vi "Config GUI - Insert Into Virtual Folder.vi"(8 "error in":errorcluster, 10 "Virtual Folder Search Output":T1, 11 "GUI Objects":T2) -> (0 "error out":errorcluster)   [LabVIEW 2022 SP3]
doc: "Configures the GUI objects that play a part in the functionality that inserts the newly created VI or CTL into a Virtual Folder."
uses:
  GUI Objects (cluster).ctl
  DFS Output (cluster).ctl
panel:
  # "Development\ncontrols/indicators useful for development and testing, but which are not outputs of the VI"
  # "Input\nInputs to the VI"
  # "Output\nOutputs of the VI"
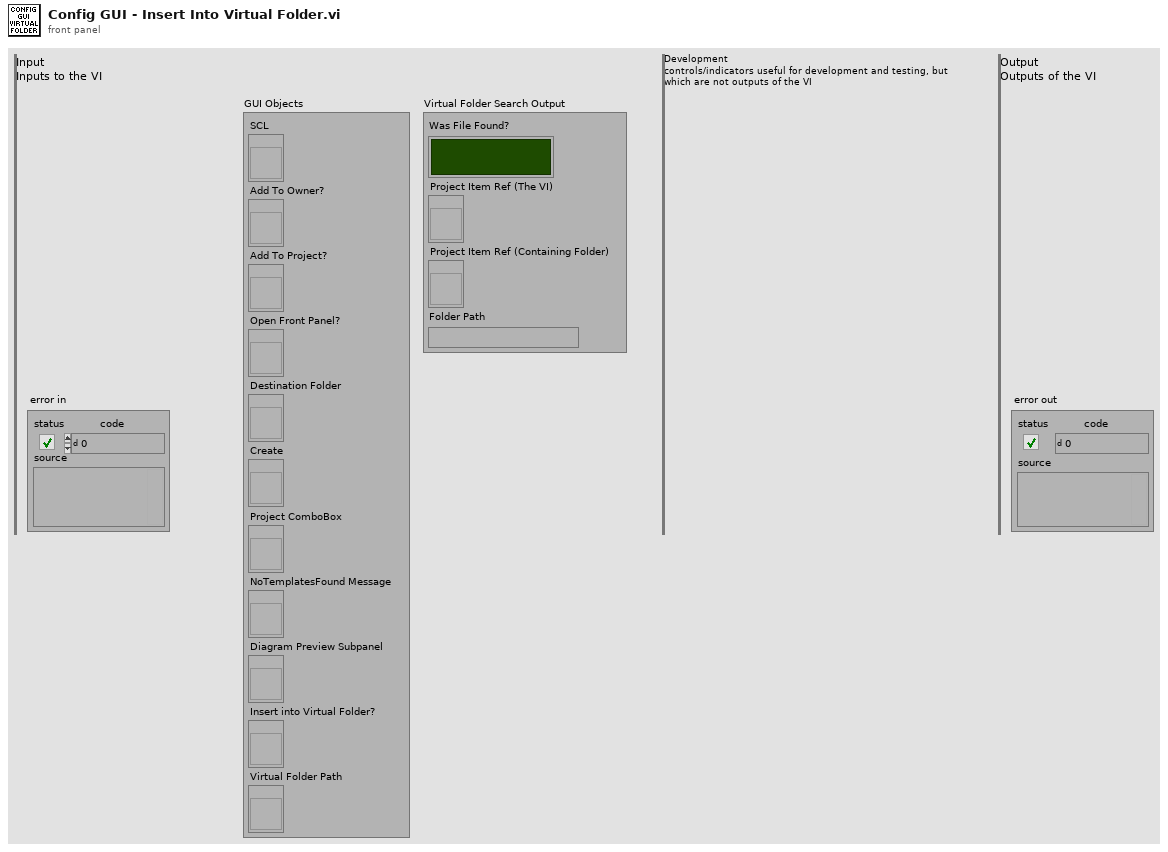
[diagram p1: front panel]
types:
  T1 = typedef "DFS Output (cluster).ctl" = cluster{"Was File Found?":bool, "Project Item Ref (The VI)":refnum<vi>, "Project Item Ref (Containing Folder)":refnum<vi>, "Folder Path":string}
  T2 = typedef "GUI Objects (cluster).ctl" = cluster{"SCL":refnum<vi>, "Add To Owner?":refnum<vi>, "Add To Project?":refnum<vi>, "Open Front Panel?":refnum<vi>, "Destination Folder":refnum<vi>, "Create":refnum<vi>, "Project ComboBox":refnum<vi>, "NoTemplatesFound Message":refnum<vi>, "Diagram Preview Subpanel":refnum<vi>, "Insert into Virtual Folder?":refnum<vi>, "Virtual Folder Path":refnum<vi>}
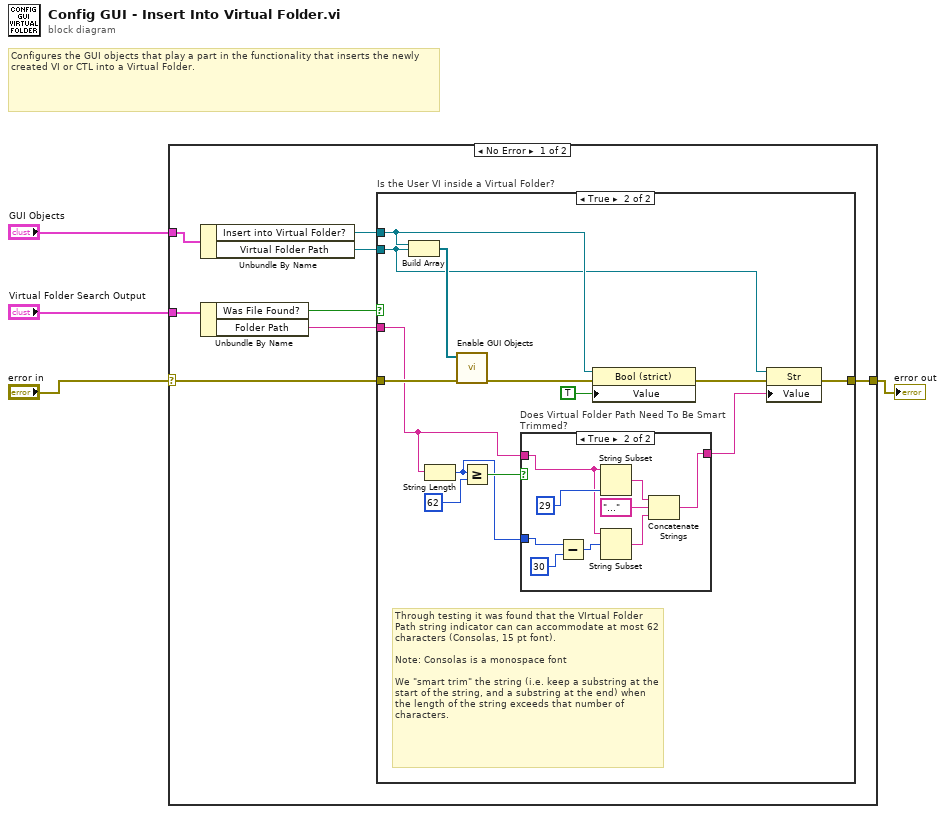
[diagram p0: block diagram]
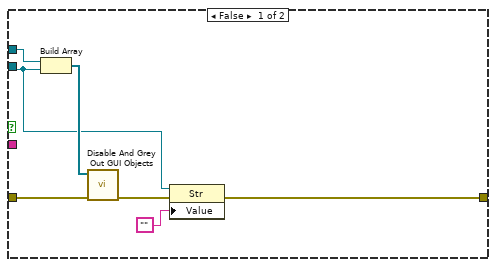
[diagram p2: hidden frame]
diagram:
  # "Configures the GUI objects that play a part in the functionality that inserts the newly created VI or CTL into a Virtual Folder."
  n1 = case shown="No Error" "error in" {
    selector: "error in" -> [w11 w43]
    tunnel: [w10 w43] -> w3
    tunnel: "GUI Objects" -> [w8 _]
    tunnel: "Virtual Folder Search Output" -> [w12 _]
    frame No Error {
      n2 = Unbundle By Name(w8) -> ("Insert into Virtual Folder?"=w7:refnum<vi>, "Virtual Folder Path"=w6:refnum<vi>)
      n3 = Unbundle By Name(w12) -> ("Was File Found?"=w9:bool, "Folder Path"=w5:string)
      n4 = case "Is the User VI inside a Virtual Folder?" shown="True" w9 {
        tunnel: w11 -> [w19 w32]
        tunnel: [w15 w26] -> w10
        tunnel: w7 -> [w16 w28]
        tunnel: w6 -> [w14 w25]
        tunnel: w5 -> [_ w22]
        frame False {
          n5 = Build Array(w16, w14) -> (w17:refnum<vi>[])
          n6 = call "Disable And Grey Out GUI Objects.vi"("Error In"=w19, "GUI Object Refs"=w17) -> ("Error Out"=w18:errorcluster)  [unwired: 9 in]
          n7 = property class="Str"(reference=w14, error in=w18, "Value"="") -> (error out=w15:errorcluster)  [unwired: 1 out]
        }
        frame True {
          # "Through testing it was found that the VIrtual Folder Path string indicator can can accommodate at most 62 characters (Consolas, 15 pt font).\n\nNote: Consolas is a monospace font\n\nWe \"smart trim\" the string (i.e. keep a substring at the start of the string, and a substring at the end) when the length of the string exceeds that number of characters."
          n8 = Build Array(w28, w25) -> (w30:refnum<vi>[])
          n9 = String Length(string=w22) -> (length=w20:i32)
          n10 = call "Enable GUI Objects.vi"("Error In"=w32, "GUI Object Refs"=w30) -> ("Error Out"=w31:errorcluster)  [unwired: 9 in]
          n11 = Greater Or Equal?(x=w20, y=62) -> (x >= y?=w23:bool)
          n12 = case "Does Virtual Folder Path Need To Be Smart Trimmed?" shown="True" w23 {
            tunnel: w22 -> [w33 w35]
            tunnel: [w33 w34] -> w21
            tunnel: w20 -> [_ w38]
            frame False {
            }
            frame True {
              n13 = Subtract(x=w38, y=30) -> (x-y=w37:i32)
              n14 = String Subset(string=w35, length (rest)=29 ("length (rest)")) -> (substring=w41:string)  [unwired: 1 in]
              n15 = String Subset(string=w35, offset (0)=w37) -> (substring=w39:string)  [unwired: 1 in]
              n16 = Concatenate Strings(w41, "..." ("string"), w39) -> (w34:string)
            }
          }
          n17 = property class="Bool (strict)"(reference=w28, error in=w31, "Value"=TRUE) -> (error out=w29:errorcluster)  [unwired: 1 out]
          n18 = property class="Str"(reference=w25, error in=w29, "Value"=w21) -> (error out=w26:errorcluster)  [unwired: 1 out]
        }
      }
    }
    frame Error {
    }
  }
  "error out" <- w3
